vi "SearchConnectedTerminals_Scripting.vi"() -> ()   [LabVIEW 2018]
uses:
  <vilib>/Utility/traverseref.llb/TRef TravTarget.ctl
  <vilib>/Utility/Data Type/Type Definitions/Data Type.ctl
  <vilib>/Utility/traverseref.llb/VI Scripting - Traverse.lvlib
  <vilib>/Utility/Data Type/NI_Data Type.lvlib
panel:
  out "Array 2":i32[](array[numeric])
  out "Array":string[][](array[string])
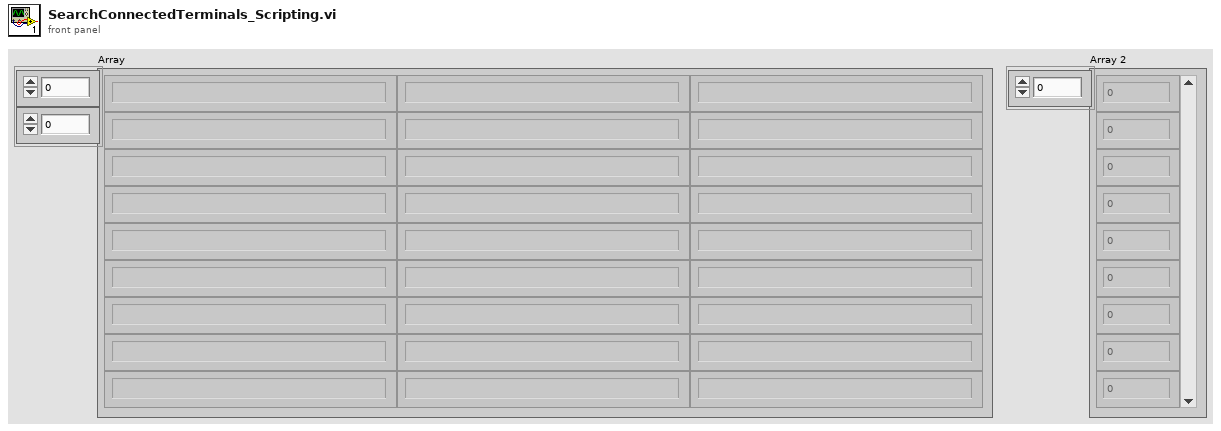
[diagram p1: front panel]
types:
  T1 = typedef "TRef TravTarget.ctl" = enum16{"FP", "BD", "Other"}
  T2 = typedef "imagedata.ctl" = cluster{"image type":i32, "image depth":i32, "image":u8[], "mask":u8[], "colors":u32[], "Rectangle":cluster{"left":i16, "top":i16, "right":i16, "bottom":i16}}
  T3 = typedef "NI_Data Type.lvlib/Data Type.ctl" = enum8{"Invalid Type", "Void", "I8", "I16", "I32", "I64", "U8", "U16", "U32", "U64", "Single Float", "Double Float", "Extended Float", "Single Complex", "Double Complex", "Extended Complex", "Enum U8", "Enum U16", "Enum U32", "Enum U64", "Single Float With Unit", "Double Float With Unit", "Extended Float With Unit", "Single Complex with Unit", "Double Complex with Unit", "Extended Complex with Unit", "Boolean", "String", "Path", "Picture", "Tag", "Array", "Cluster", "Variant", "LV Variant", "Waveform", "Timestamp", "Digital Waveform", "Digital Data", "ExpressData", "Refnum", "External Data", "VI", "Poly VI", "LabVIEW Class Instance", "Fixed Point"}
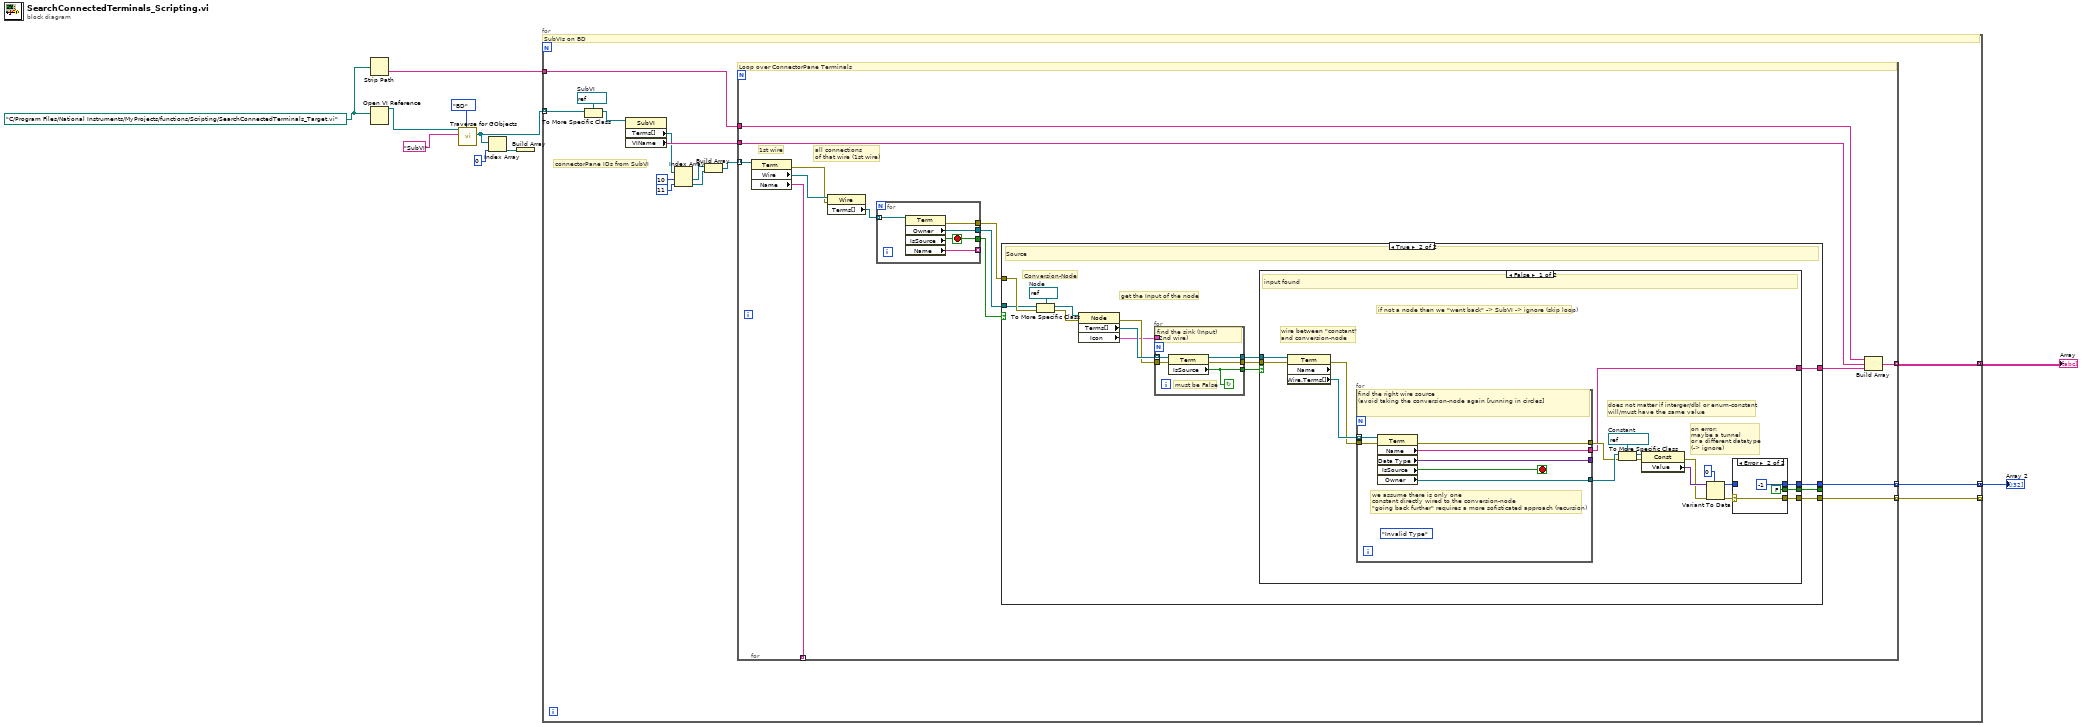
[diagram p0: block diagram]
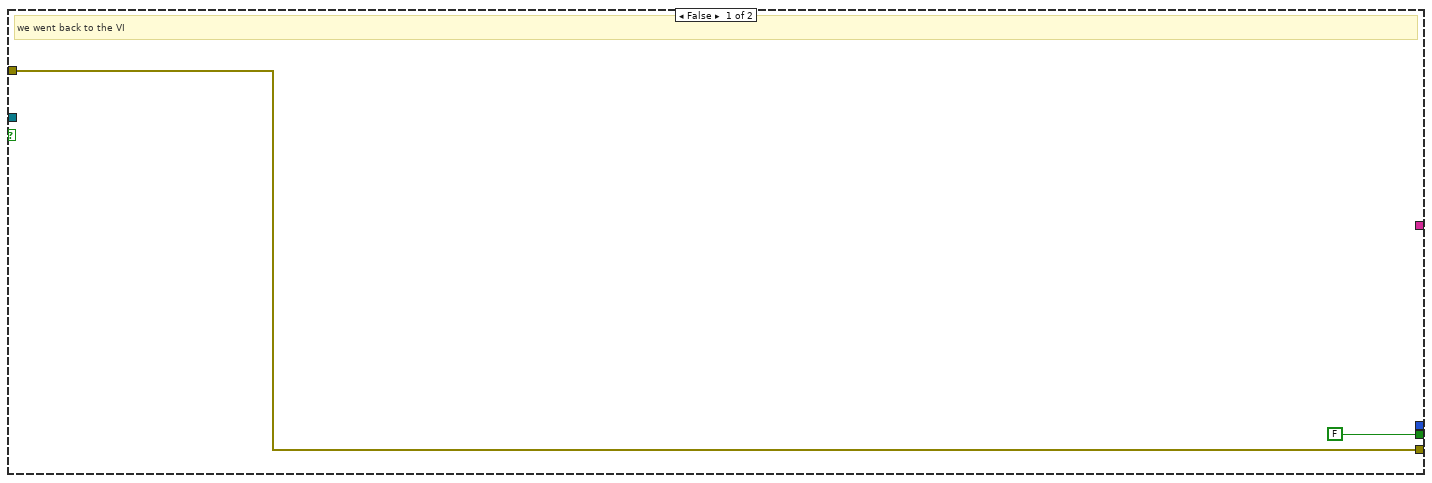
[diagram p2: hidden frame]
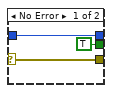
[diagram p3: hidden frame]
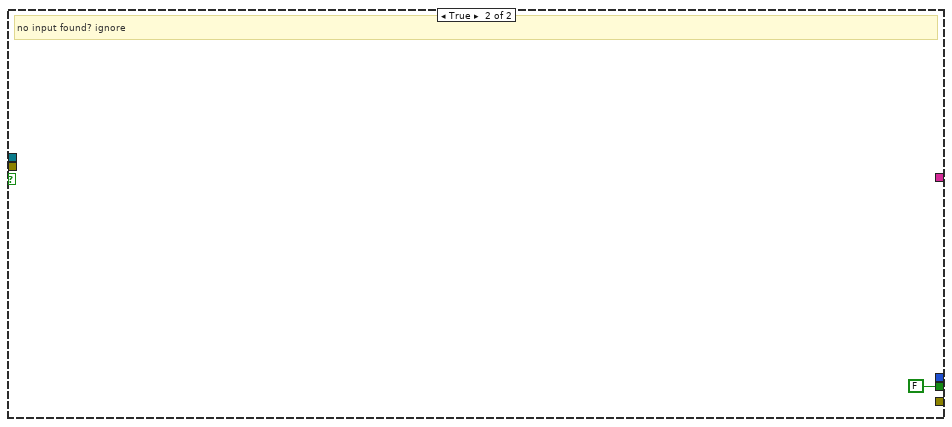
[diagram p4: hidden frame]
diagram:
  w3 = path "C:/Program Files/National Instruments/MyProjects/functions/Scripting/SearchConnectedTerminals_Target.vi" ("vi path")
  n1 = Strip Path(path=w3) -> (name=w2:string)  [unwired: 1 out]
  n2 = Open VI Reference(vi path=w3) -> (vi reference=w10:refnum<vi>)  [unwired: 5 in, 1 out]
  n3 = call <vilib>:"Traverse for GObjects.vi"("Traverse Target"=TRef_TravTarget."BD", "Class Name"="SubVI", "VI Refnum"=w10) -> ("References"=w5:refnum<vi>[])  [unwired: 5 in, 3 out]
  n4 = Index Array(array=w5, index=0) -> (element=w6:refnum<vi>)
  n5 = Build Array(w6) -> ()  [unwired: 1 out]
  n6 = for {
    tunnel: w5 -> [w24] mode=indexing
    tunnel: [w11] -> w4 mode=concatenating
    tunnel: [w14] -> w1 mode=concatenating
    tunnel: [w13] -> _ mode=indexing
    tunnel: w2 -> [w12]
    w23 = refnum<vi> refnum  # SubVI
    # "connectorPane IDs from SubVI"
    # "SubVIs on BD"
    n7 = To More Specific Class(target class=w23, reference=w24) -> (specific class reference=w22:refnum<vi>)  [unwired: 1 in, 1 out]
    n8 = property class="SubVI"(reference=w22) -> ("Terms[]"=w20:refnum<vi>[], "VIName"=w21:string)  [unwired: 1 in, 2 out]
    n9 = Index Array(array=w20, index #1=10 ("index"), index #2=11 ("index")) -> (element #1=w19:refnum<vi>, element #2=w18:refnum<vi>)
    n10 = Build Array(w19, w18) -> (w17:refnum<vi>[])
    n11 = for {
      tunnel: w17 -> [w38] mode=indexing
      tunnel: w21 -> [w32]
      tunnel: [w36] -> _ mode=indexing
      tunnel: [w35] -> w14 mode=indexing
      tunnel: [w33] -> w13 mode=indexing
      tunnel: w12 -> [w30]
      tunnel: [w31] -> w11 mode=indexing
      # "all connections\nof that wire (1st wire)"
      # "1st wire"
      # "Loop over ConnectorPane Terminals"
      n12 = property class="Term"(reference=w38) -> (error out=w34:errorcluster, "Wire"=w37:refnum<vi>, "Name"=w36:string)  [unwired: 1 in, 1 out]
      n13 = property class="Wire"(reference=w37, error in=w34) -> ("Terms[]"=w29:refnum<vi>[])  [unwired: 2 out]
      n14 = for {
        tunnel: w29 -> [w97] mode=indexing
        tunnel: [w96] -> w28
        tunnel: [w95] -> w27
        tunnel: [w94] -> _ mode=indexing
        tunnel: [w93] -> w26
        stop <- w95 stop-if-true
        n15 = property class="Term"(reference=w97) -> (error out=w96:errorcluster, "Owner"=w93:refnum<vi>, "IsSource"=w95:bool, "Name"=w94:string)  [unwired: 1 in, 1 out]
      }
      n16 = case shown="True" w27 {
        tunnel: [_ w53] -> w25
        tunnel: [_ w52] -> w35
        tunnel: w28 -> [w40 w51]
        tunnel: [w40 w44] -> w33
        tunnel: [FALSE w42] -> _
        tunnel: w26 -> [_ w41]
        frame False {
          # "we went back to the VI"
        }
        frame True {
          w55 = refnum<vi> refnum  # Node
          # "get the Input of the node"
          # "Conversion-Node"
          # "Source"
          n17 = To More Specific Class(target class=w55, reference=w41, error in=w51) -> (specific class reference=w54:refnum<vi>, error out=w50:errorcluster)
          n18 = property class="Node"(reference=w54, error in=w50) -> (error out=w47:errorcluster, "Terms[]"=w49:refnum<vi>[], "Icon"=w43:T2)  [unwired: 1 out]
          n19 = for {
            tunnel: w49 -> [w92] mode=indexing
            tunnel: [w91] -> w48
            tunnel: w47 -> [w90]
            tunnel: [w89] -> w46
            tunnel: [w88] -> w45
            tunnel: w43 -> [_]
            stop <- w88 continue-if-true
            # "must be False"
            # "find the sink (Input)\n(2nd wire)"
            n20 = property class="Term"(reference=w92, error in=w90) -> (reference out=w91:refnum<vi>, error out=w89:errorcluster, "IsSource"=w88:bool)
          }
          n21 = case shown="False" w45 {
            tunnel: [w56 _] -> w53
            tunnel: [w58 _] -> w52
            tunnel: w48 -> [w65 _]
            tunnel: w46 -> [w64 _]
            tunnel: [w61 _] -> w44
            tunnel: [w59 FALSE] -> w42
            frame False {
              w72 = refnum<vi> refnum  # Constant
              # "if not a node then we \"went back\" -> SubVI -> ignore (skip loop)"
              # "on error:\nmaybe a tunnel\nor a different datatype\n(-> ignore)"
              # "does not matter if interger/dbl or enum-constant\nwill/must have the same value"
              # "wire between \"constant\"\nand conversion-node"
              # "input found"
              n22 = property class="Term" props=["Name", "Wire", "Terms[]"](reference=w65, error in=w64) -> (error out=w66:errorcluster, "Wire.Terms[]"=w73:refnum<vi>[])  [unwired: 2 out]
              n23 = for {
                tunnel: [w86] -> w56
                tunnel: w73 -> [w85] mode=indexing
                tunnel: [w84] -> _
                tunnel: [w82] -> w70
                tunnel: w66 -> [w80]
                tunnel: [w81] -> w62
                stop <- w83 stop-if-true
                (unwired) Data_Type."Invalid Type" ("Type")
                # "we assume there is only one\nconstant directly wired to the conversion-node\n\"going back further\" requires a more sofisticated approach (recursion)"
                # "find the right wire source\n(avoid taking the conversion-node again [running in circles]"
                n24 = property class="Term"(reference=w85, error in=w80) -> (error out=w81:errorcluster, "Name"=w86:string, "Data Type"=w84:variant, "IsSource"=w83:bool, "Owner"=w82:refnum<vi>)  [unwired: 1 out]
              }
              n25 = To More Specific Class(target class=w72, reference=w70, error in=w62) -> (specific class reference=w71:refnum<vi>, error out=w67:errorcluster)
              n26 = property class="Const"(reference=w71, error in=w67) -> (error out=w63:errorcluster, "Value"=w69:variant)  [unwired: 1 out]
              n27 = Variant To Data(error in=w63, type=0, Variant=w69) -> (data=w57:i32, error out=w60:errorcluster)
              n28 = case shown="Error" w60 {
                selector: w60 -> [w76 w78]
                tunnel: [w76 w78] -> w61
                tunnel: [TRUE FALSE] -> w59
                tunnel: [w74 -1] -> w58
                tunnel: w57 -> [w74 _]
                frame No Error {
                }
                frame Error {
                }
              }
            }
            frame True {
              # "no input found? ignore"
            }
          }
        }
      }
      n29 = Build Array(w30, w32, w25) -> (w31:string[])
    }
  }
  "Array" <- w4
  "Array 2" <- w1
